vi "FitLorentzian.vi"(10 "y":dbl[](array[numeric]), 11 "x":dbl[](array[numeric])) -> (3 "best fit parameters":dbl[](array[numeric]) caption="pos\nwidth\nheight\noffset" format="%.4e")   [LabVIEW 2017]
uses:
  <vilib>/Analysis/baseanly.llb/Mean (DBL).vi
  <vilib>/gmath/NumericalOptimization/Nonlinear Curve Fit LM.vi
  <vilib>/gmath/NI_Gmath.lvlib
  <vilib>/Analysis/NI_AALBase.lvlib
panel:
  out "Parameter Guess":dbl[](array[numeric]) caption="pos\nwidth\namplitude*\noffset" format="%.4e"
  out "XY Graph":cluster{cdb[]}[](graph)
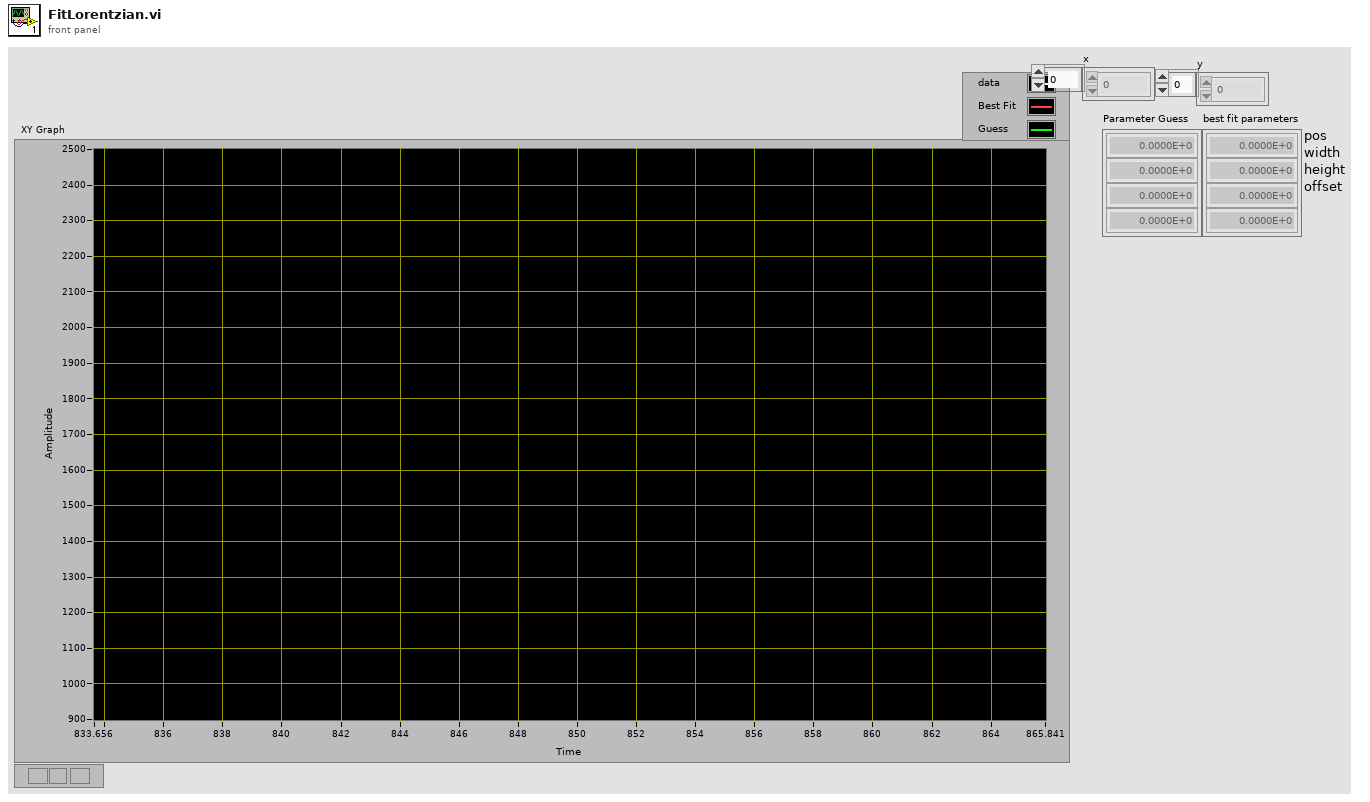
[diagram p1: front panel]
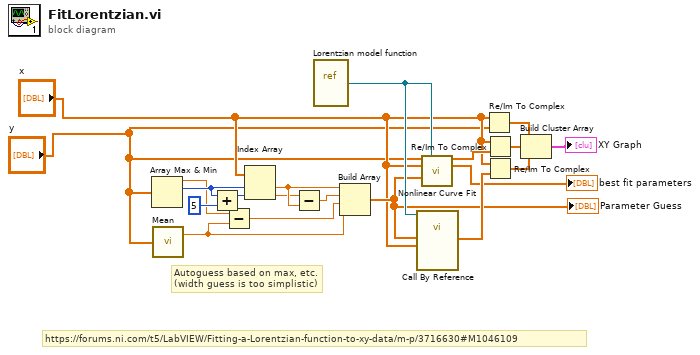
[diagram p0: block diagram]
diagram:
  # "https://forums.ni.com/t5/LabVIEW/Fitting-a-Lorentzian-function-to-xy-data/m-p/3716630#M1046109"
  # "Autoguess based on max, etc.\n(width guess is too simplistic)"
  n1 = Array Max & Min(array="y") -> (max value=w5:dbl, max index (indices)=w19:i32)  [unwired: 2 out]
  n2 = call-poly <vilib>:"Mean.vi"("X"="y") -> ("mean"=w6:dbl)  [unwired: 1 out]
  n3 = Add(x=w19, y=5) -> (x+y=w18:i32)
  n4 = Subtract(x=w5, y=w6) -> (x-y=w3:dbl)
  n5 = Index Array(array="x", index #1=w19, index #2=w18) -> (element #1=w16:dbl, element #2=w15:dbl)
  n6 = Subtract(x=w15, y=w16) -> (x-y=w13:dbl)
  n7 = vi-ref "Lorentzian model function.vi"() -> (w12:refnum<vi>)
  n8 = Build Array(w16, w13, w3, w6) -> (w4:dbl[])
  "Parameter Guess" <- w4
  n9 = call-by-ref "?"(reference=w12, "X"="x", "a"=w4) -> ("f(X,a)"=w10:dbl[])  [unwired: 3 in, 4 out]
  n10 = call-poly <vilib>:"Nonlinear Curve Fit.vi"("Y"="y", "f(x,a)"=w12, "X"="x", "initial parameters"=w4) -> ("best nonlinear fit"=w8:dbl[], "best fit parameters"=→"best fit parameters":dbl[])  [unwired: 6 in, 4 out]
  n11 = Re/Im To Complex(1:"y", 2:"x") -> (0:w20:cdb[])
  n12 = Re/Im To Complex(1:w8, 2:"x") -> (0:w11:cdb[])
  n13 = Re/Im To Complex(1:w10, 2:"x") -> (0:w9:cdb[])
  n14 = Build Cluster Array(w20, w11, w9) -> (→"XY Graph":cluster{cdb[]}[])
